vi "G#Debugger_UpdateAttributes.vi"(0 "Objects dvr":refnum<data-value>, 1 "Subpanel dvr":refnum<data-value>, 2 "tag":string, 3 "class attributes":bool, 4 "inheritance index":i32, 5 "error in (no error)":errorcluster) -> (12 "string":string, 14 "Only read attributes":bool, 15 "attributes reference":refnum<vi>, 16 "attributes value":variant, 17 "valid object":bool, 18 "# of users?":i32, 19 "error out":errorcluster)   [LabVIEW 2020, in "G#Debugger.lvlib"]
uses:
  <vilib>/addons/_AddQ/G#Debugger/G#Debugger.lvlib
  <vilib>/addons/_AddQ/G#Object/utils/G#Object_ClassInfoType.ctl
  <vilib>/addons/_AddQ/G#Object/G#Object.lvclass
  <vilib>/addons/_AddQ/G#Object/utils/G#Object_ObjectInfoType.ctl
  <vilib>/addons/_AddQ/G#Object/utils/G#Object_CreateMethod.ctl
  <vilib>/addons/_AddQ/G#Debugger/private/G#Debugger_SubPanelInfo.ctl
  <vilib>/addons/_AddQ/G#Object/utils/G#Object_ClassHierarchy.ctl
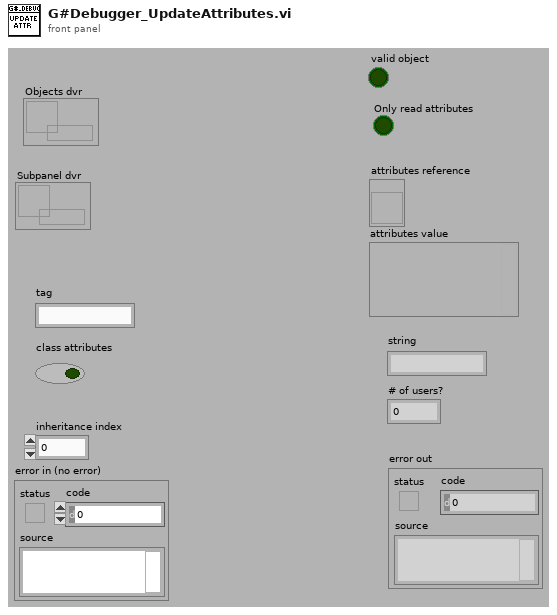
[diagram p1: front panel]
types:
  T1 = typedef "G#Debugger.lvlib/G#Debugger_SubPanelInfo.ctl" = cluster{"Ref":refnum<class "G#Object.lvclass">, "class hierarchy":T2[], "class attributes":path[], "object attributes":path[], "inheritance index":i32, "is class attributes":bool, "vi reference":refnum<vi>}
  T2 = typedef "G#Object.lvclass/G#Object_ClassHierarchy.ctl" = cluster{"ClassName":string, "FullClassName":string, "ClassPath":path, "IsLeaf":bool}
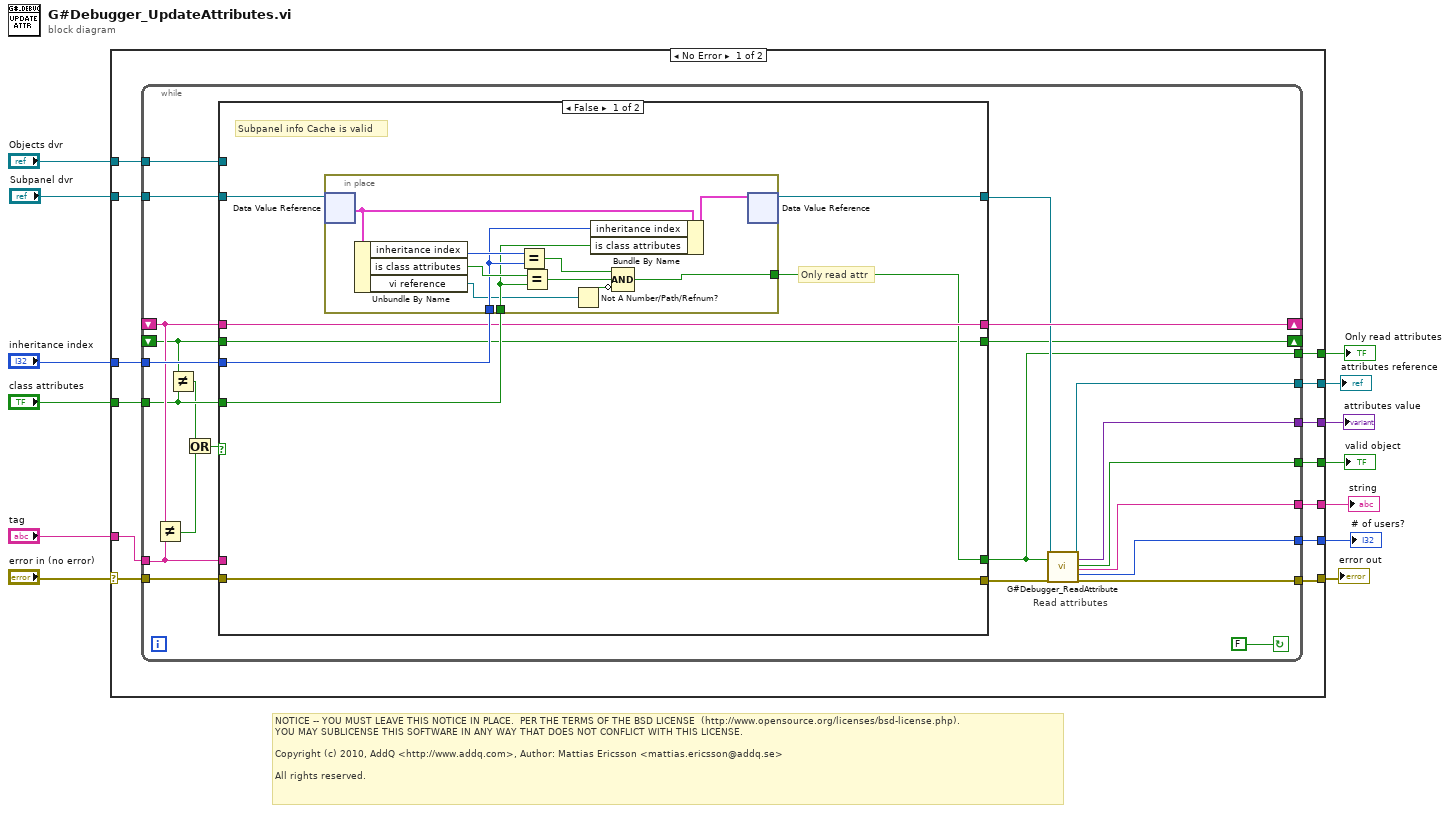
[diagram p0: block diagram]
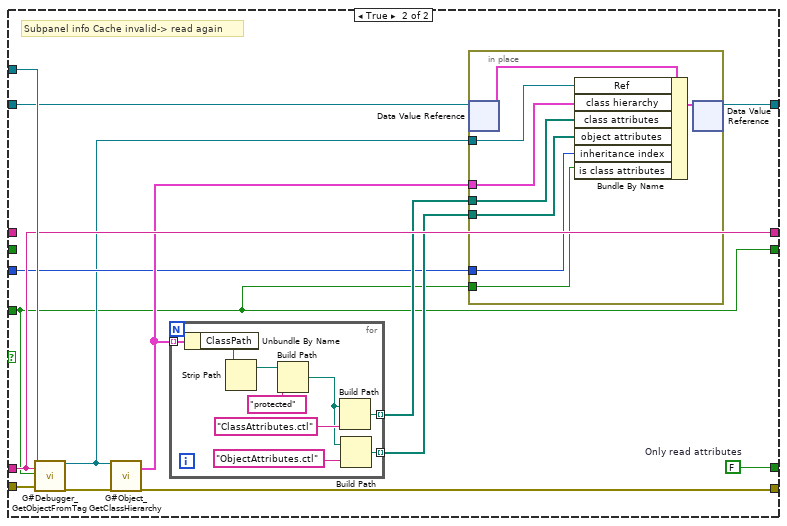
[diagram p2: hidden frame]
diagram:
  # "NOTICE -- YOU MUST LEAVE THIS NOTICE IN PLACE.  PER THE TERMS OF THE BSD LICENSE  (http://www.opensource.org/licenses/bsd-license.php).\nYOU MAY SUBLICENSE THIS SOFTWARE IN ANY WAY THAT DOES NOT CONFLICT WITH THIS LICENSE.\n\nCopyright (c) 2010, AddQ <http://www.addq.com>, Author: Mattias Ericsson <mattias.ericsson@addq.se>\n\nAll rights reserved."
  n1 = case shown="No Error" "error in (no error)" {
    selector: "error in (no error)" -> [w23 w100]
    tunnel: [w20 w100] -> w12
    tunnel: "inheritance index" -> [w26 _]
    tunnel: "class attributes" -> [w25 _]
    tunnel: "tag" -> [w24 _]
    tunnel: "Objects dvr" -> [w22 _]
    tunnel: "Subpanel dvr" -> [w21 _]
    tunnel: [w19 _] -> w6
    tunnel: [w18 _] -> w5
    tunnel: [w17 _] -> w4
    tunnel: [w16 _] -> w3
    tunnel: [w15 _] -> w2
    tunnel: [w14 _] -> w1
    frame No Error {
      n2 = while {
        tunnel: w26 -> [w49]
        tunnel: w25 -> [w31]
        tunnel: w24 -> [w46]
        tunnel: w23 -> [w48]
        tunnel: w22 -> [w47]
        shift-right: [w43] -> _
        shift-left: _ -> [w45]
        tunnel: w21 -> [w44]
        tunnel: [w39] -> w20
        tunnel: [w38] -> w19
        tunnel: [w37] -> w18
        tunnel: [w36] -> w17
        tunnel: [w35] -> w16
        tunnel: [w34] -> w15
        tunnel: [w33] -> w14
        shift-right: [w32] -> _
        shift-left: _ -> [w30]
        stop <- FALSE continue-if-true
        # "Read attributes"
        n3 = Not Equal?(x=w45, y=w46) -> (x != y?=w28:bool)
        n4 = Not Equal?(x=w30, y=w31) -> (x != y?=w29:bool)
        n5 = Or(x=w29, y=w28) -> (x .or. y?=w27:bool)
        n6 = case shown="False" w27 {
          tunnel: w49 -> [w55 w73]
          tunnel: w31 -> [w54 w69]
          tunnel: w48 -> [w57 w82]
          tunnel: w47 -> [_ w81]
          tunnel: w46 -> [_ w80]
          tunnel: [w53 w80] -> w43
          tunnel: w45 -> [w53 _]
          tunnel: [w57 w78] -> w41
          tunnel: w44 -> [w56 w77]
          tunnel: [w52 w72] -> w40
          tunnel: [w51 w71] -> w36
          tunnel: w30 -> [w50 _]
          tunnel: [w50 w69] -> w32
          frame False {
            # "Only read attr"
            # "Subpanel info Cache is valid"
            n7 = in-place {
              in-place-border: w55 -> [w64]
              in-place-border: w54 -> [w63]
              in-place-border: [w60] -> w51
              n8 = in-place-dvr #1(w56) -> (w67:T1)  [unwired: 1 out]
              n9 = Unbundle By Name(w67) -> ("inheritance index"=w66:i32, "is class attributes"=w65:bool, "vi reference"=w58:refnum<vi>)
              n10 = Equal?(x=w66, y=w64) -> (x = y?=w62:bool)
              n11 = Equal?(x=w65, y=w63) -> (x = y?=w61:bool)
              n12 = Not A Number/Path/Refnum?(number/path/refnum=w58) -> (NaN/Path/Refnum?=w59:bool)
              n13 = Bundle By Name(cluster=w67, "inheritance index"=w64, "is class attributes"=w63) -> (w68:T1)
              n14 = Compound Arithmetic op=AND(w62, w61, invert w59) -> (w60:bool)
              n15 = in-place-dvr #1(w68) -> (w52:refnum<data-value>)  [unwired: 1 out]
            }
          }
          frame True {
            w71 = FALSE  # Only read attributes
            # "Subpanel info Cache invalid-> read again"
            n16 = call <vilib>:"G#Debugger_GetObjectFromTag.vi"("Objects dvr"=w81, "Tag"=w80, "class attributes"=w69, "error in (no error)"=w82) -> ("Ref"=w70:refnum<class "G#Object.lvclass">, "error out"=w79:errorcluster)  [unwired: 13 in, 1 out]
            n17 = call <vilib>:"G#Object_GetClassHierarchy.vi"("reference in"=w70, "error in (no error)"=w79) -> ("class hierarchy"=w76:T2[], "error out"=w78:errorcluster)  [unwired: 15 in, 1 out]
            n18 = for {
              tunnel: w76 -> [w99] mode=indexing
              tunnel: [w96] -> w75 mode=indexing
              tunnel: [w95] -> w74 mode=indexing
              n19 = Unbundle By Name(w99) -> ("ClassPath"=w94:path)
              n20 = Strip Path(path=w94) -> (stripped path=w93:path)  [unwired: 1 out]
              n21 = Build Path(base path=w93, name or relative path="protected") -> (appended path=w92:path)
              n22 = Build Path(base path=w92, name or relative path="ClassAttributes.ctl") -> (appended path=w96:path)
              n23 = Build Path(base path=w92, name or relative path="ObjectAttributes.ctl") -> (appended path=w95:path)
            }
            n24 = in-place {
              in-place-border: w70 -> [w90]
              in-place-border: w76 -> [w88]
              in-place-border: w75 -> [w87]
              in-place-border: w74 -> [w86]
              in-place-border: w73 -> [w85]
              in-place-border: w69 -> [w84]
              n25 = in-place-dvr #2(w77) -> (w83:T1)  [unwired: 1 out]
              n26 = Bundle By Name(cluster=w83, "Ref"=w90, "class hierarchy"=w88, "class attributes"=w87, "object attributes"=w86, "inheritance index"=w85, "is class attributes"=w84) -> (w89:T1)
              n27 = in-place-dvr #2(w89) -> (w72:refnum<data-value>)  [unwired: 1 out]
            }
          }
        }
        n28 = call <vilib>:"G#Debugger_ReadAttribute.vi"("Subpanel dvr"=w40, "Only read attributes"=w36, "error in (no error)"=w41) -> ("attributes reference"=w38:refnum<vi>, "attributes value"=w37:variant, "valid object"=w35:bool, "string"=w34:string, "# of users?"=w33:i32, "error out"=w39:errorcluster)  [unwired: 11 in]
      }
    }
    frame Error {
    }
  }
  "error out" <- w12
  "attributes reference" <- w6
  "attributes value" <- w5
  "Only read attributes" <- w4
  "valid object" <- w3
  "string" <- w2
  "# of users?" <- w1
